vi "Revision Query.vi"(0 "VISA resource name":refnum<visa-resource-name>, 11 "error in (no error)":errorcluster) -> (4 "VISA resource name out":refnum<visa-resource-name>, 6 "Instrument Driver Revision":string, 8 "Instrument Firmware Revision":string, 10 "Instrument Model":string, 15 "error out":errorcluster)   [LabVIEW 2020, in "NH Research Regenerative Test Series.lvlib"]
uses:
  NH Research Regenerative Test Series.lvlib
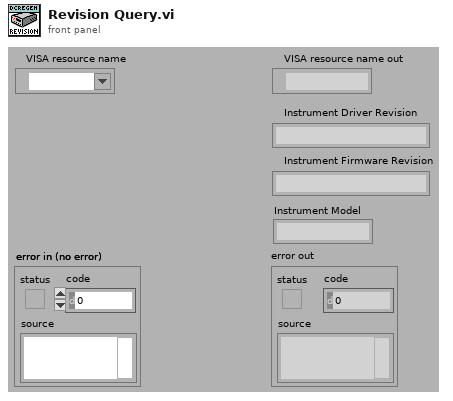
[diagram p1: front panel]
types:
  T1 = cluster{"Major":u16, "Minor":u16, "Fix":u16, "Build":u16}
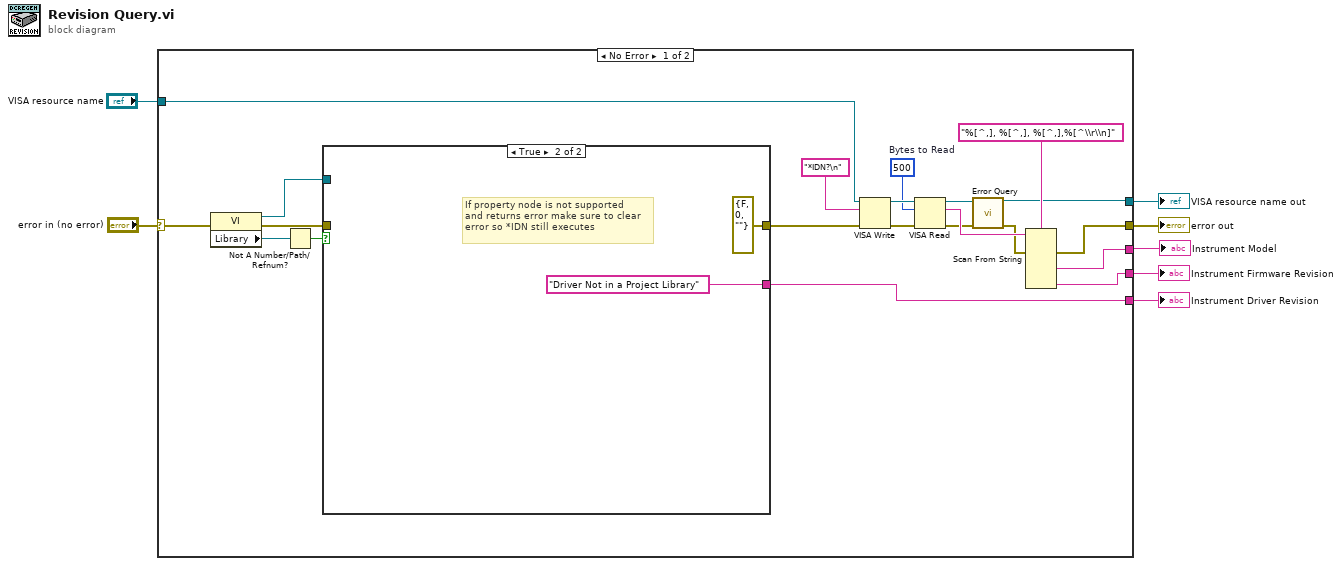
[diagram p0: block diagram]
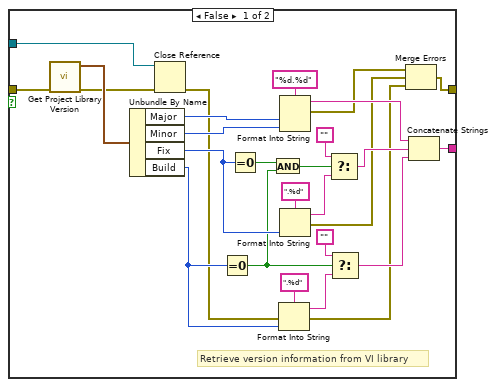
[diagram p2: hidden frame]
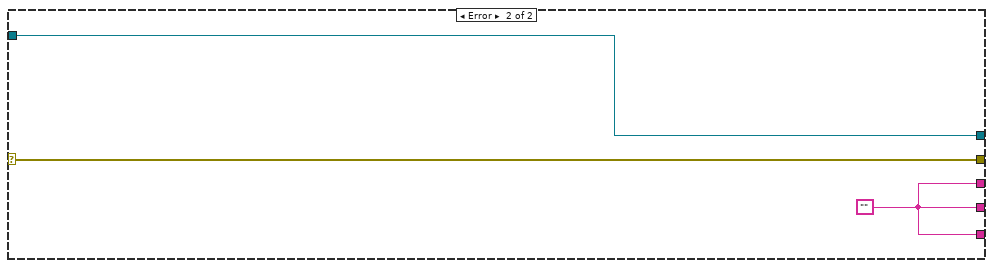
[diagram p3: hidden frame]
diagram:
  n1 = case shown="No Error" "error in (no error)" {
    selector: "error in (no error)" -> [w12 w60]
    tunnel: "VISA resource name" -> [w28 w59]
    tunnel: [w20 w58] -> w2
    tunnel: [w16 w59] -> w6
    tunnel: [w13 w60] -> w1
    tunnel: [w21 w58] -> w5
    tunnel: [w18 w58] -> w3
    frame No Error {
      w22 = u32 500  # Bytes to Read
      n2 = property on="Property Node" class="VI"(error in=w12) -> (reference out=w11:refnum<vi>, error out=w10:errorcluster, "Library"=w9:refnum<vi>)  [unwired: 1 in]
      n3 = Not A Number/Path/Refnum?(number/path/refnum=w9) -> (NaN/Path/Refnum?=w8:bool)
      n4 = case shown="True" w8 {
        tunnel: w11 -> [w55 _]
        tunnel: w10 -> [w31 _]
        tunnel: [w32 errorcluster {"status"=FALSE, "code"=0, "source"=""} ("error IO")] -> w23
        tunnel: [w37 "Driver Not in a Project Library"] -> w21
        frame False {
          # "Retrieve version information from VI library"
          n5 = call "Get Project Library Version.vi"("error in (no error)"=w31) -> ("error out"=w29:errorcluster, "Project Library Version"=w30:T1)  [unwired: 9 in]
          n6 = Unbundle By Name(w30) -> ("Major"=w44:u16, "Minor"=w43:u16, "Fix"=w41:u16, "Build"=w42:u16)
          n7 = Close Reference(reference=w55, error in (no error)=w29) -> (error out=w36:errorcluster)
          n8 = Equal To 0?(x=w42) -> (x = 0?=w39:bool)
          n9 = Equal To 0?(x=w41) -> (x = 0?=w40:bool)
          n10 = And(x=w40, y=w39) -> (x .and. y?=w38:bool)
          n11 = Format Into String(format string=".%d", error in=w36, w42) -> (resulting string=w48:string, error out=w33:errorcluster)  [unwired: 1 in]
          n12 = Format Into String(format string="%d.%d", w44, w43) -> (resulting string=w50:string, error out=w35:errorcluster)  [unwired: 2 in]
          n13 = Format Into String(format string=".%d", w41) -> (resulting string=w52:string, error out=w34:errorcluster)  [unwired: 2 in]
          n14 = Select(t="" ("Empty String Constant"), s=w38, f=w52) -> (s? t:f=w49:string)
          n15 = Select(t="" ("Empty String Constant"), s=w39, f=w48) -> (s? t:f=w45:string)
          n16 = Merge Errors(w35, w34, w33) -> (w32:errorcluster)
          n17 = Concatenate Strings(w50, w49, w45) -> (w37:string)
        }
        frame True {
          # "If property node is not supported\nand returns error make sure to clear\nerror so *IDN still executes"
        }
      }
      n18 = VISA Write(VISA resource name=w28, write buffer="*IDN?\n", error in (no error)=w23) -> (VISA resource name out=w27:refnum<visa-resource-name>, error out=w26:errorcluster)  [unwired: 1 out]
      n19 = VISA Read(VISA resource name=w27, byte count=w22, error in (no error)=w26) -> (VISA resource name out=w17:refnum<visa-resource-name>, read buffer=w19:string, error out=w15:errorcluster)  [unwired: 1 out]
      n20 = call "Error Query.vi"("VISA resource name"=w17, "error in (no error)"=w15) -> ("VISA resource name out"=w16:refnum<visa-resource-name>, "error out"=w14:errorcluster)  [unwired: 10 in, 2 out]
      n21 = Scan From String(format string="%[^,], %[^,], %[^,],%[^\\r\\n]", input string=w19, error in=w14) -> (error out=w13:errorcluster, output 2=w18:string, output 4=w20:string)  [unwired: 7 in, 2 out]
    }
    frame Error {
      w58 = "" ("Empty String Constant")
    }
  }
  "Instrument Firmware Revision" <- w2
  "Instrument Driver Revision" <- w5
  "VISA resource name out" <- w6
  "error out" <- w1
  "Instrument Model" <- w3
